vi "GetInheritance_DEPRECATED.vi"(0 "LibReader in":refnum<class "LibReader.lvclass">, 5 "error in (no error)":errorcluster) -> (14 "LibReader out":refnum<class "LibReader.lvclass">, 15 "Inheritance":path[](array[path]), 16 "Inherits":bool, 19 "error out":errorcluster)   [LabVIEW 2014]
uses:
  <resource>/Framework/Providers/Open_GDS/ClassProviders/LibProvider_BaseClassInterface/LibReader_class/LibReader.lvclass
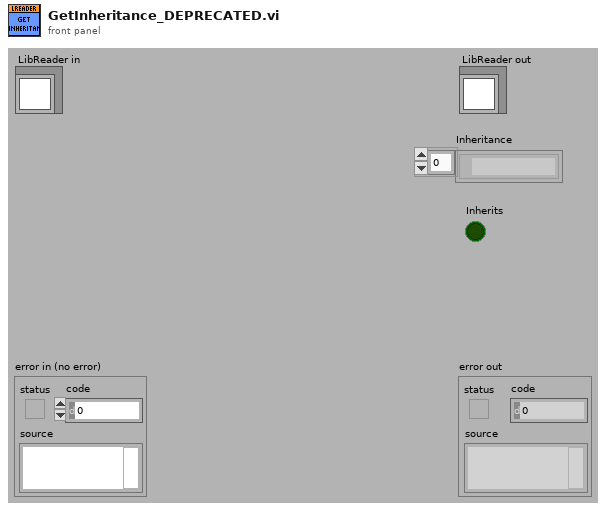
[diagram p1: front panel]
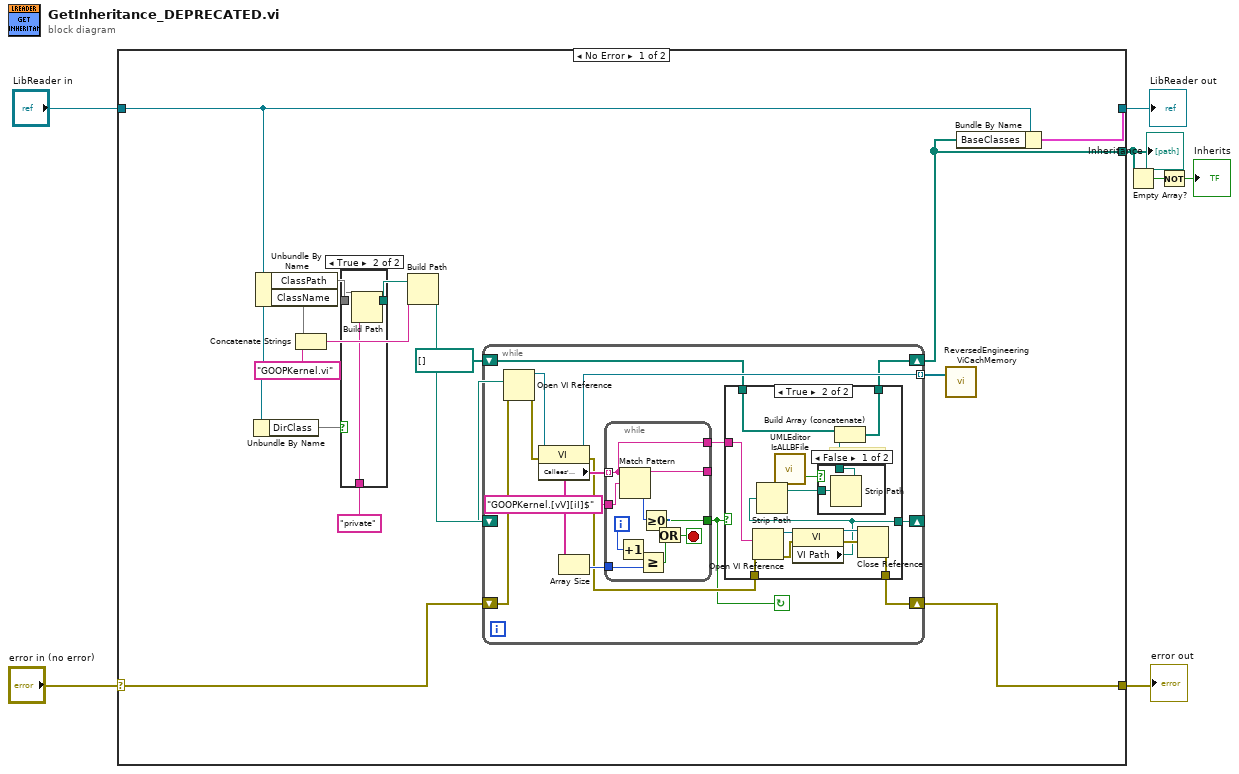
[diagram p0: block diagram]
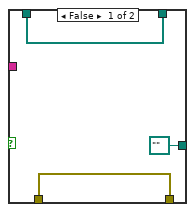
[diagram p3: hidden frame]
diagram:
  n1 = case shown="No Error" "error in (no error)" {
    selector: "error in (no error)" -> [w13 w72]
    tunnel: [w12 w72] -> w6
    tunnel: [w9 w71] -> w4
    tunnel: "LibReader in" -> [w10 w71]
    tunnel: [w8 _] -> w3
    frame No Error {
      n2 = Unbundle By Name(w10) -> ("DirClass"=w18)
      n3 = Unbundle By Name(w10) -> ("ClassPath"=w19, "ClassName"=w14)
      n4 = Concatenate Strings(w14, "GOOPKernel.vi" ("string")) -> (w16:string)
      n5 = case shown="True" w18 {
        tunnel: w19 -> [w23 w26]
        tunnel: [w23 w25] -> w20
        tunnel: "private" ("element") -> [_ w24]
        frame False {
        }
        frame True {
          n6 = Build Path(base path=w26, name or relative path=w24) -> (appended path=w25:path)
        }
      }
      n7 = Build Path(base path=w20, name or relative path=w16) -> (appended path=w17:path)
      n8 = while {
        shift-right: [w32] -> w12
        shift-left: w13 -> [w34]
        tunnel: [w31] -> w22 mode=indexing
        shift-right: [w29] -> _
        shift-left: w17 -> [w30]
        shift-right: [w27] -> w8
        shift-left: path[] [] -> [w28]
        stop <- w33 continue-if-true
        n9 = Open VI Reference(vi path=w30, error in (no error)=w34) -> (vi reference=w41:refnum<vi>, error out=w40:errorcluster)  [unwired: 4 in]
        n10 = property class="VI"(reference=w41, error in=w40) -> (reference out=w31:refnum<vi>, error out=w35:errorcluster, "Callees' Names"=w39:string[])
        n11 = Array Size(array=w39) -> (size(s)=w37:i32)
        n12 = while {
          tunnel: w39 -> [w63] mode=indexing
          tunnel: "GOOPKernel.[vV][iI]$" ("string") -> [w70]
          tunnel: w37 -> [w61]
          tunnel: [w65] -> w33
          tunnel: [w64] -> _
          tunnel: [w63] -> w36
          i -> [w69]
          stop <- w66 stop-if-true
          n13 = Increment(x=w69) -> (x+1=w62:i32)
          n14 = Match Pattern(string=w63, regular expression=w70) -> (before substring=w64:string, offset past match=w68:i32)  [unwired: 1 in, 2 out]
          n15 = Greater Or Equal?(x=w62, y=w61) -> (x >= y?=w67:bool)
          n16 = Greater Or Equal To 0?(x=w68) -> (x >= 0?=w65:bool)
          n17 = Or(x=w65, y=w67) -> (x .or. y?=w66:bool)
        }
        n18 = case shown="True" w33 {
          tunnel: w36 -> [_ w57]
          tunnel: w35 -> [w44 w52]
          tunnel: [w44 w51] -> w32
          tunnel: w28 -> [w43 w45]
          tunnel: [w43 w46] -> w27
          tunnel: [path "" ("Path") w50] -> w29
          frame False {
          }
          frame True {
            # "Iheritance"
            n19 = Open VI Reference(vi path=w57, error in (no error)=w52) -> (vi reference=w56:refnum<vi>, error out=w55:errorcluster)  [unwired: 4 in]
            n20 = property class="VI"(reference=w56, error in=w55) -> (reference out=w54:refnum<vi>, error out=w53:errorcluster, "VI Path"=w50:path)
            n21 = Strip Path(path=w50) -> (stripped path=w48:path)  [unwired: 1 out]
            n22 = call <resource>:"UMLEditor IsALLBFile.vi"("path"=w48) -> ("path to VI library?"=w49:bool)
            n23 = case shown="False" w49 {
              tunnel: [w58 w60] -> w47
              tunnel: w48 -> [w59 w60]
              frame False {
                n24 = Strip Path(path=w59) -> (stripped path=w58:path)  [unwired: 1 out]
              }
              frame True {
              }
            }
            n25 = Build Array (concatenate)(w45, w47) -> (w46:path[])
            n26 = Close Reference(reference=w54, error in (no error)=w53) -> (error out=w51:errorcluster)
          }
        }
      }
      n27 = call <resource>:"ReversedEngineering ViCachMemory.vi"("ViRef-Array"=w22) -> ()  [unwired: 18 in, 1 out]
      n28 = Bundle By Name(cluster=w10, "BaseClasses"=w8) -> (w9:cluster{})
    }
    frame Error {
    }
  }
  "error out" <- w6
  "LibReader out" <- w4
  "Inheritance" <- w3
  n29 = Empty Array?(array=w3) -> (empty?=w2:bool)
  n30 = Not(x=w2) -> (.not. x?=→"Inherits":bool)
